vi "Post-Build Action.vi"(5 "Files Generated by Build":path[](array[path]), 6 "Top Level/Always Included VIs":path[](array[path]), 7 "Destination Path":path, 8 "error in (no error)":errorcluster, 9 "Target Name":string, 10 "Build Specification Name":string, 11 "Project Path":path) -> (0 "error out":errorcluster)   [LabVIEW 2017]
uses:
  <userlib>/_OpenG.lib/lvzip/lvzip.llb/ZLIB Open ZIP Mode__ogtk.ctl
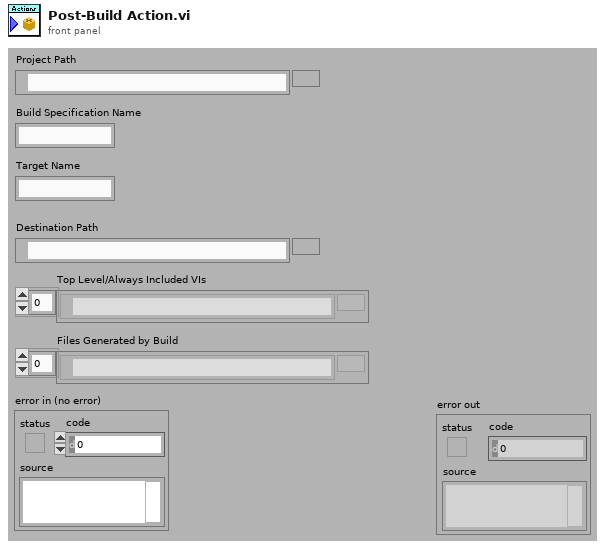
[diagram p1: front panel]
types:
  T1 = typedef "ZLIB Open ZIP Mode__ogtk.ctl" = enum16{"create new", "append to end", "append to archive"}
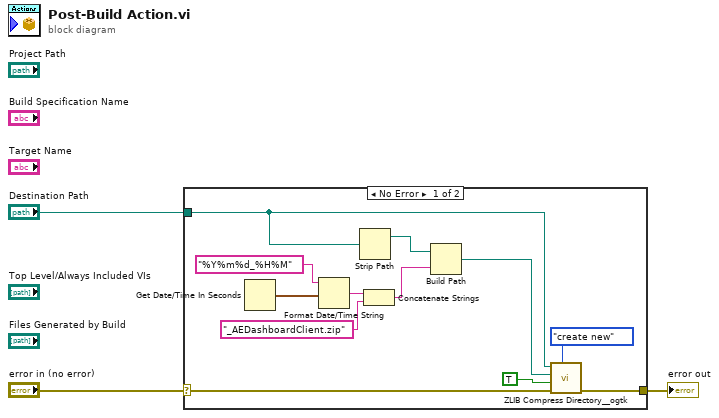
[diagram p0: block diagram]
diagram:
  n1 = case shown="No Error" "error in (no error)" {
    selector: "error in (no error)" -> [w9 w16]
    tunnel: [w4 w16] -> w2
    tunnel: "Destination Path" -> [w6 _]
    frame No Error {
      n2 = Get Date/Time In Seconds() -> (seconds since 1Jan1904=w14:timestamp)
      n3 = Format Date/Time String(time format string (%c)="%Y%m%d_%H%M", seconds (now)=w14) -> (date/time string=w12:string)  [unwired: 1 in]
      n4 = Strip Path(path=w6) -> (stripped path=w15:path)  [unwired: 1 out]
      n5 = Concatenate Strings(w12, "_AEDashboardClient.zip") -> (w10:string)
      n6 = Build Path(base path=w15, name or relative path=w10) -> (appended path=w7:path)
      n7 = call <userlib>:"ZLIB Compress Directory__ogtk.vi"("append (create new)"=ZLIB_Open_ZIP_Mode__ogtk."create new", "error in (no error)"=w9, "include subdirectories (F)"=TRUE, "archive name (root directory with .zip ending)"=w7, "root directory (file dialog)"=w6) -> ("error out"=w4:errorcluster)  [unwired: 4 in, 2 out]
    }
    frame Error {
    }
  }
  "error out" <- w2
